vi "ActorDatabase-PerformInsertInstruction.vi"(8 "error in (no error)":errorcluster, 11 "Database-Actor in":refnum<class "Database-Actor.lvclass">=refnum) -> (0 "error out":errorcluster, 3 "Database-Actor out":refnum<class "Database-Actor.lvclass">)   [LabVIEW 2013, in "Database-Actor.lvclass"]
uses:
  Database-Actor.lvclass
  Reuse Library/Database API/Database-API.lvclass
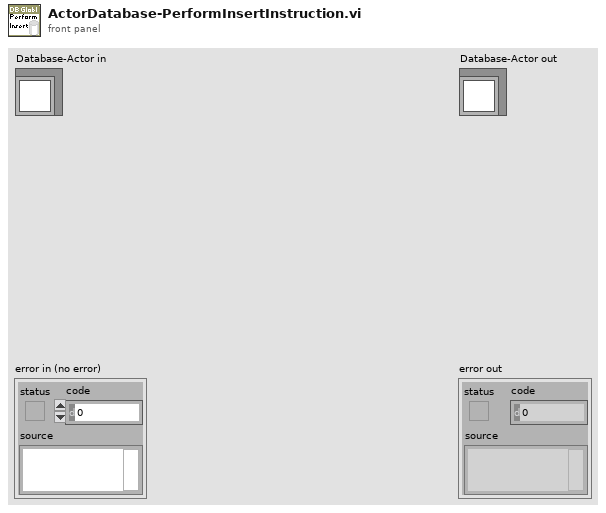
[diagram p1: front panel]
types:
  T1 = cluster{"Table":string, "SQL Statement":string, "Update All":bool, "Payload":string, "Reply Command":string}
  T2 = cluster{"Manufacturing-Part Number":string, string, "Label Instructions":string, "Path for Picture Label":path, "Path for Picture Label 2":path, "Path for Picture Label 3":path, "Path for Picture Label 4":path, "Path for Picture Label 5":path, "Path for Picture Label 6":path, "Path for Picture Label 7":path, "General Instruction Name":string}[]
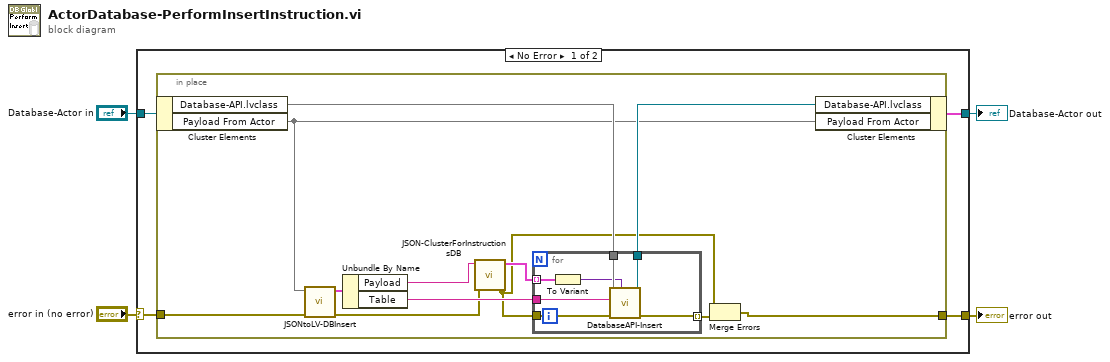
[diagram p0: block diagram]
diagram:
  n1 = case shown="No Error" "error in (no error)" {
    selector: "error in (no error)" -> [w8 w29]
    tunnel: [w7 w29] -> w3
    tunnel: [w5 w28] -> w1
    tunnel: "Database-Actor in" -> [w6 w28]
    frame No Error {
      n2 = in-place {
        in-place-border: w8 -> [w17]
        in-place-border: [w9] -> w7
        n3 = in-place-cluster #1(w6) -> ("Database-API.lvclass"=w20, "Payload From Actor"=w18)
        n4 = call "JSONtoLV-DBInsert.vi"("error in"=w17, "Output JSON Object"=w18) -> ("error out"=w13:errorcluster, "value"=w16:T1)  [unwired: 8 in]
        n5 = Unbundle By Name(w16) -> ("Payload"=w14:string, "Table"=w15:string)
        n6 = call "JSON-ClusterForInstructionsDB.vi"("error in (no error)"=w13, "Payload"=w14) -> ("error out"=w10:errorcluster, "Cluster Out"=w12:T2)  [unwired: 8 in]
        n7 = for {
          tunnel: w20 -> [w27]
          tunnel: [w26] -> w19
          tunnel: w15 -> [w25]
          tunnel: w10 -> [w24]
          tunnel: [w23] -> w11 mode=indexing
          tunnel: w12 -> [w22] mode=indexing
          n8 = To Variant(anything=w22) -> (Variant=w21:variant)
          n9 = call "DatabaseAPI-Insert.vi"("Cluster Data for DB"=w21, "error in (no error)"=w24, "Table"=w25, "Database-API in"=w27) -> ("error out"=w23:errorcluster, "Database-API out"=w26:refnum<class "Database-API.lvclass">)  [unwired: 6 in]
        }
        n10 = Merge Errors(w10, w11) -> (w9:errorcluster)
        n11 = in-place-cluster #1("Database-API.lvclass"=w19, "Payload From Actor"=w18) -> (w5:cluster{})
      }
    }
    frame Error {
    }
  }
  "error out" <- w3
  "Database-Actor out" <- w1
